vi "update.description.request.vi"(8 "error in":errorcluster, 11 "description":string) -> (0 "error out":errorcluster, 1 "Request":string)   [LabVIEW 2020, in "asset.lvclass"]
uses:
  116a1f63-1174-4f6f-bedf-07de5800daec.vi
  <vilib>/JDP Science/JSONtext/Variant to JSON Text.vi
  <vilib>/JDP Science/JSONtext/LVClass Serializer/JSONtext LVClass Serializer.lvclass
  asset.lvclass
  asset.lvclass/asset.ctl
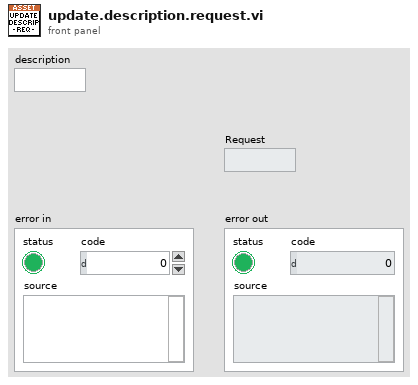
[diagram p1: front panel]
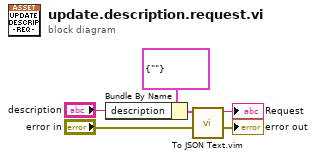
[diagram p0: block diagram]
diagram:
  n1 = Bundle By Name(cluster=cluster{"description":string} {"description"=""}, "description"="description") -> (w5:cluster{"description":string})
  n2 = call "To JSON Text.vim"("error in (no error)"="error in", "Anything"=w5) -> ("error out"=→"error out":errorcluster, "<JSON>"=→"Request":string)  [unwired: 8 in]
